vi "GetLVHandlers.vi"(1 "Server":T2) -> (0 "Handlers":T1)   [LabVIEW 2017]
uses:
  <vilib>/WebServerConfig/Server.ctl
  <vilib>/WebServerConfig/Alias.ctl
  <vilib>/WebServerConfig/ErrorDocument.ctl
  <vilib>/WebServerConfig/Action.ctl
  <vilib>/WebServerConfig/Redirect.ctl
  <vilib>/WebServerConfig/Interface.ctl
  <vilib>/WebServerConfig/AddHandler.ctl
  <vilib>/WebServerConfig/SSL.ctl
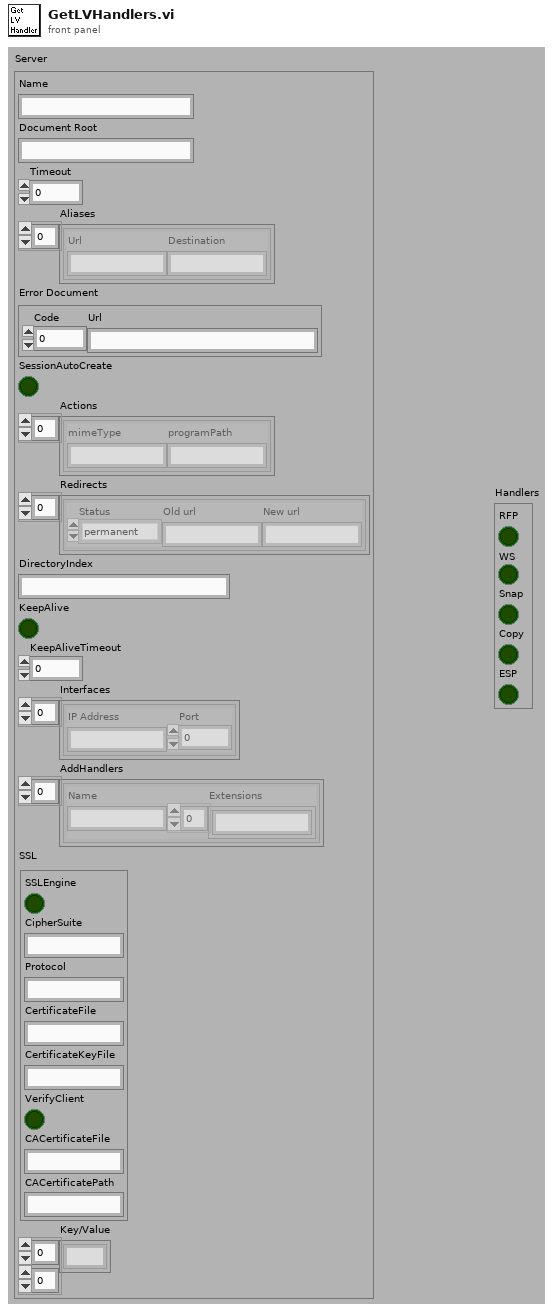
[diagram p1: front panel]
types:
  T1 = cluster{"RFP":bool, "WS":bool, "Snap":bool, "Copy":bool, "ESP":bool}
  T2 = typedef "Server.ctl" = cluster{"Name":string, "Document Root":string, "Timeout":u32, "Aliases":T3[], "Error Document":T4, "SessionAutoCreate":bool, "Actions":T5[], "Redirects":T6[], "DirectoryIndex":string, "KeepAlive":bool, "KeepAliveTimeout":u32, "Interfaces":T7[], "AddHandlers":T8[], "SSL":T9, "Key/Value":string[][]}
  T3 = typedef "Alias.ctl" = cluster{"Url":string, "Destination":string}
  T4 = typedef "ErrorDocument.ctl" = cluster{"Code":u16, "Url":string}
  T5 = typedef "Action.ctl" = cluster{"mimeType":string, "programPath":string}
  T6 = typedef "Redirect.ctl" = cluster{"Status":enum16{"permanent", "temp", "seeother", "gone"}, "Old url":string, "New url":string}
  T7 = typedef "Interface.ctl" = cluster{"IP Address":string, "Port":u16}
  T8 = typedef "AddHandler.ctl" = cluster{"Name":string, "Extensions":string[]}
  T9 = typedef "SSL.ctl" = cluster{"SSLEngine":bool, "CipherSuite":string, "Protocol":string, "CertificateFile":string, "CertificateKeyFile":string, "VerifyClient":bool, "CACertificateFile":string, "CACertificatePath":string}
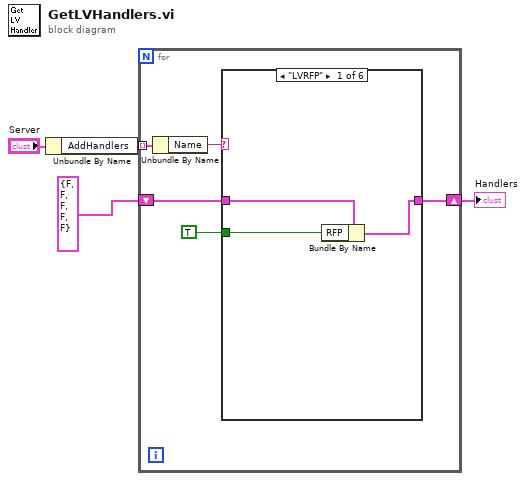
[diagram p0: block diagram]
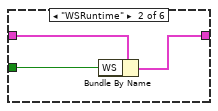
[diagram p2: hidden frame]
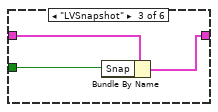
[diagram p3: hidden frame]
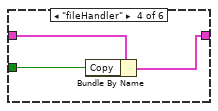
[diagram p4: hidden frame]
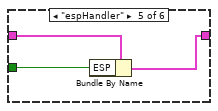
[diagram p5: hidden frame]
diagram:
  n1 = Unbundle By Name("Server") -> ("AddHandlers"=w3:T8[])
  n2 = for {
    tunnel: w3 -> [w9] mode=indexing
    shift-right: [w7] -> w1
    shift-left: T1 {"RFP"=FALSE, "WS"=FALSE, "Snap"=FALSE, "Copy"=FALSE, "ESP"=FALSE} ("Handlers") -> [w6]
    n3 = Unbundle By Name(w9) -> ("Name"=w8:string)
    n4 = case shown="\"LVRFP\"" w8 {
      tunnel: [w11 w14 w16 w19 w22 w25] -> w7
      tunnel: w6 -> [w12 w15 w17 w20 w23 w25]
      tunnel: TRUE -> [w10 w13 w18 w21 w24 _]
      frame "LVRFP" {
        n5 = Bundle By Name(cluster=w12, "RFP"=w10) -> (w11:T1)
      }
      frame "WSRuntime" {
        n6 = Bundle By Name(cluster=w15, "WS"=w13) -> (w14:T1)
      }
      frame "LVSnapshot" {
        n7 = Bundle By Name(cluster=w17, "Snap"=w18) -> (w16:T1)
      }
      frame "fileHandler" {
        n8 = Bundle By Name(cluster=w20, "Copy"=w21) -> (w19:T1)
      }
      frame "espHandler" {
        n9 = Bundle By Name(cluster=w23, "ESP"=w24) -> (w22:T1)
      }
      frame Default {
      }
    }
  }
  "Handlers" <- w1
